vi "Set Amplitude_biploar.vi"(7 "Channel Name (1)":u8(ring)=1 items=["1"=1, "2"=2, "3"=3, "4"=4], 8 "error in (no error)":errorcluster, 10 "Amplitude V":dbl=1.2, 11 "VISA resource name":refnum<visa-resource-name>="GPIB0::1::INSTR") -> (0 "error out":errorcluster)   [LabVIEW 2021]
uses:
  <instrlib>/Tektronix AWG 5000 7000 Series/Tektronix AWG 5000 7000 Series.lvlib
panel:
  in  "Offset V":dbl
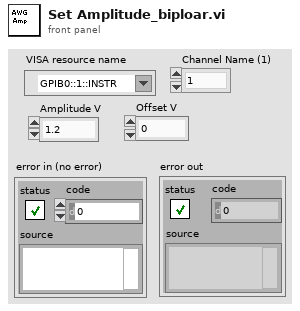
[diagram p1: front panel]
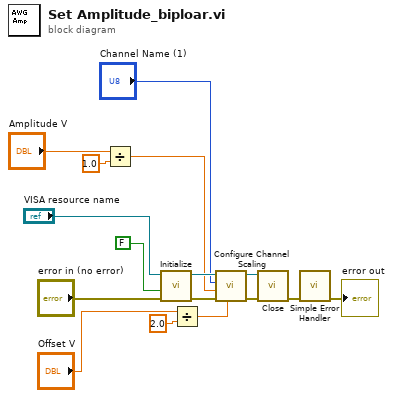
[diagram p0: block diagram]
diagram:
  n1 = Divide(x="Amplitude V", y=1.0) -> (x/y=w4:dbl)
  n2 = call <instrlib>:"Initialize.vi"("error in (no error)"="error in (no error)", "Reset (False)"=FALSE ("Reset? (F: No)"), "VISA resource name"="VISA resource name") -> ("error out"=w11:errorcluster, "VISA resource name out"=w10:refnum<visa-resource-name>)  [unwired: 7 in]
  n3 = Divide(x="Offset V", y=2.0) -> (x/y=w2:dbl)
  n4 = call <instrlib>:"Configure Channel Scaling.vi"("Offset (0 V)"=w2, "error in (no error)"=w11, "Amplitude (0.5 Vpp)"=w4, "Channel Name (1)"="Channel Name (1)", "VISA resource name"=w10) -> ("error out"=w8:errorcluster, "VISA resource name out"=w9:refnum<visa-resource-name>)  [unwired: 5 in]
  n5 = call <instrlib>:"Close.vi"("error in (no error)"=w8, "VISA resource name"=w9) -> ("error out"=w13:errorcluster)  [unwired: 9 in]
  n6 = call <vilib>:"Simple Error Handler.vi"("error in (no error)"=w13) -> ("error out"=→"error out":errorcluster)  [unwired: 4 in, 4 out]
